vi "Example Graph.vi"() -> ()   [LabVIEW 2013]
uses:
  C:/tf/play/labview/Tinkerforge.dll
  Tinkerforge.dll
panel:
  in  "semsor identifier":u8=179
  in  "stop":bool
  out "graph":sgl[](graph)
  in  "uid":string="Fax"
  in  "port":i32=4223
  in  "host":string="localhost"
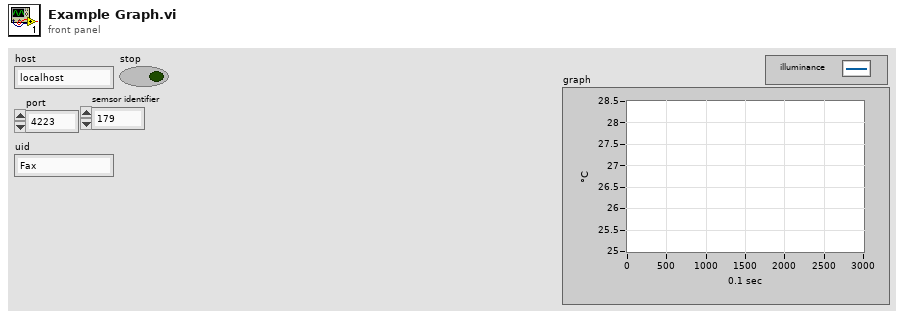
[diagram p1: front panel]
types:
  T1 = cluster{"humidity":u8, "identifier":u8, "temperature":i16}
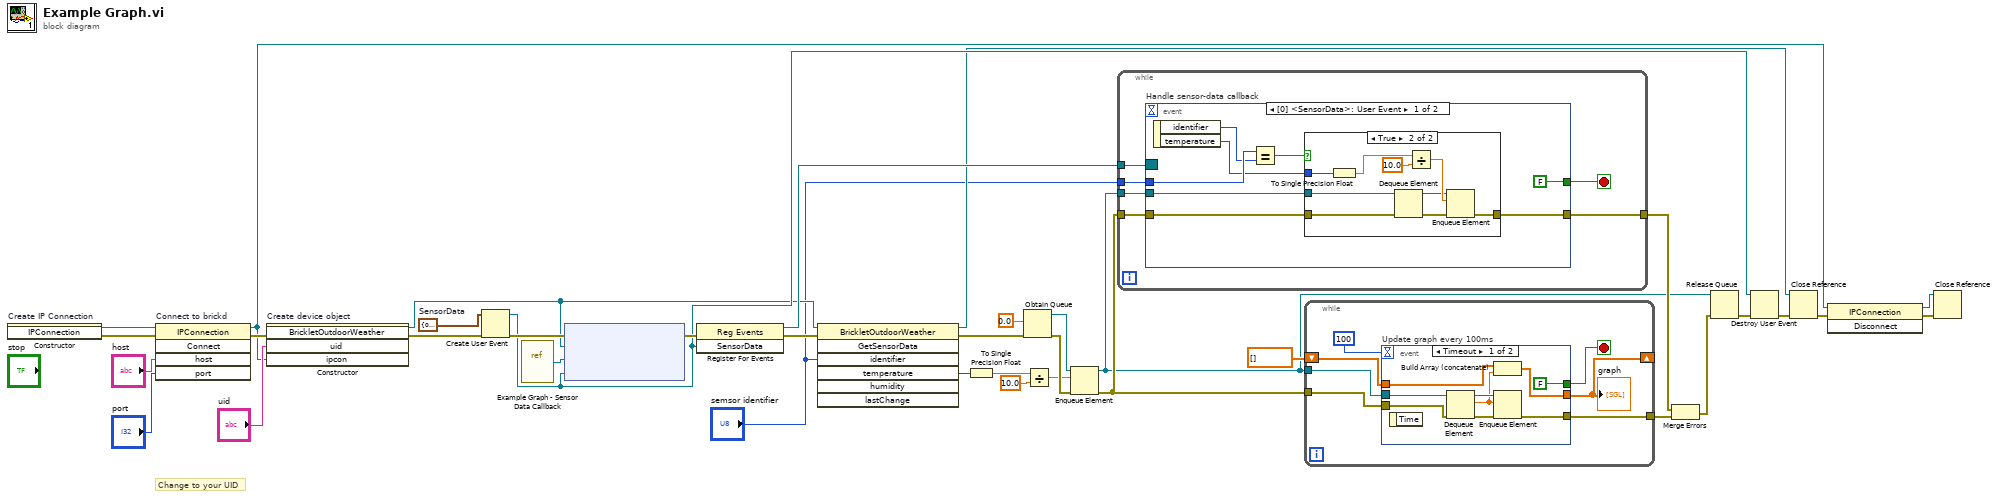
[diagram p0: block diagram]
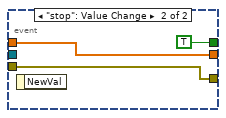
[diagram p2: hidden frame]
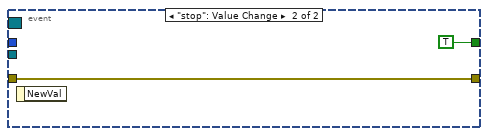
[diagram p4: hidden frame]
diagram:
  w23 = T1 {"humidity"=0, "identifier"=0, "temperature"=0}  # SensorData
  # "Change to your UID"
  n1 = constructor on="Create IP Connection" class="IPConnection"() -> (reference out=w37:refnum<k24>, error out=w12:errorcluster)  [unwired: 3 in, 1 out]
  n2 = invoke on="Connect to brickd" class="IPConnection" method="Connect"(reference=w37, error in=w12, "host"="host", "port"="port") -> (reference out=w30:refnum<k24>, error out=w33:errorcluster)  [unwired: 1 in, 3 out]
  n3 = constructor on="Create device object" class="BrickletOutdoorWeather"(error in=w33, "uid"="uid", "ipcon"=w30) -> (reference out=w6:refnum<k24>, error out=w5:errorcluster)  [unwired: 2 in, 3 out]
  n4 = Create User Event(user event datatype=w23, error in=w5) -> (user event=w25:refnum<user-event>, error out=w28:errorcluster)
  n5 = vi-ref "Example Graph - Sensor Data Callback.vi"() -> ("vi reference"=w4:refnum<vi>)
  n6 = node ("Register Event Callback")(w28, w6, w4, w25) -> (w27:errorcluster)  [unwired: 1 in, 1 out]
  n7 = register-events(error in=w27, w25) -> (reference out=w26:refnum<event-registration>, error out=w11:errorcluster)  [unwired: 1 in]
  n8 = invoke class="BrickletOutdoorWeather" method="GetSensorData"(reference=w6, error in=w11, "identifier"="semsor identifier") -> (reference out=w9:refnum<k24>, error out=w10:errorcluster, "temperature"=w2:i16)  [unwired: 4 in, 4 out]
  n9 = To Single Precision Float(number=w2) -> (single precision float=w1:sgl)
  n10 = Obtain Queue(element data type=sgl 0.0, error in (no error)=w10) -> (queue out=w16:refnum<queue>, error out=w18:errorcluster)  [unwired: 3 in, 1 out]
  n11 = Divide(x=w1, y=sgl 10.0) -> (x/y=w7:sgl)
  n12 = Enqueue Element(queue=w16, element=w7, error in (no error)=w18) -> (queue out=w13:refnum<queue>, error out=w17:errorcluster)  [unwired: 1 in, 1 out]
  n13 = while {
    tunnel: w26 -> [w43]
    tunnel: [w41] -> w21
    tunnel: w17 -> [w42]
    tunnel: w13 -> [w40]
    tunnel: "semsor identifier" -> [w38]
    stop <- w39 stop-if-true
    n14 = event "Handle sensor-data callback" shown="[0] <SensorData>: User Event" {
      selector: w43 -> [_ _]
      dyn-events: _ -> [_ _]
      timeout: _ -> [_ _]
      tunnel: w42 -> [w45 w62]
      tunnel: [w44 w62] -> w41
      tunnel: w40 -> [w46 _]
      tunnel: [FALSE TRUE] -> w39
      tunnel: w38 -> [w50 _]
      event User Event {
        n15 = event-data() -> ("identifier"=w49:u8, "temperature"=w47:i16)  [unwired: 1 in]
        n16 = Equal?(x=w50, y=w49) -> (x = y?=w48:bool)
        n17 = case shown="True" w48 {
          tunnel: w47 -> [_ w61]
          tunnel: w46 -> [_ w55]
          tunnel: w45 -> [w52 w54]
          tunnel: [w52 w53] -> w44
          frame False {
          }
          frame True {
            n18 = To Single Precision Float(number=w61) -> (single precision float=w56:sgl)
            n19 = Dequeue Element(queue=w55, error in (no error)=w54) -> (queue out=w59:refnum<queue>, error out=w58:errorcluster)  [unwired: 1 in, 2 out]
            n20 = Divide(x=w56, y=sgl 10.0) -> (x/y=w60:sgl)
            n21 = Enqueue Element(queue=w59, element=w60, error in (no error)=w58) -> (error out=w53:errorcluster)  [unwired: 1 in, 2 out]
          }
        }
      }
      event "stop": Value Change {
        n22 = event-data() -> ()  [unwired: 1 in, 1 out]
      }
    }
  }
  n23 = while {
    tunnel: [w66] -> w22
    tunnel: w17 -> [w67]
    shift-right: [w68] -> _
    shift-left: sgl[] [] -> [w69]
    tunnel: w13 -> [w65]
    stop <- w64 stop-if-true
    n24 = event "Update graph every 100ms" shown="[0] Timeout" {
      selector: _ -> [_ _]
      dyn-events: _ -> [_ _]
      timeout: 100 -> [_ _]
      tunnel: [w79 w81] -> w68
      tunnel: w69 -> [w72 w81]
      tunnel: w67 -> [w78 w80]
      tunnel: [w75 w80] -> w66
      tunnel: w65 -> [w77 _]
      tunnel: [FALSE TRUE] -> w64
      event Timeout {
        n25 = event-data() -> ()  [unwired: 1 in, 1 out]
        n26 = Dequeue Element(queue=w77, error in (no error)=w78) -> (queue out=w74:refnum<queue>, element=w73:sgl, error out=w76:errorcluster)  [unwired: 1 in, 1 out]
        n27 = Build Array (concatenate)(w72, w73) -> (w79:sgl[])
        n28 = Enqueue Element(queue=w74, element=w73, error in (no error)=w76) -> (error out=w75:errorcluster)  [unwired: 1 in, 2 out]
      }
      event "stop": Value Change {
        n29 = event-data() -> ()  [unwired: 1 in, 1 out]
      }
    }
    "graph" <- w68
  }
  n30 = Merge Errors(w21, w22) -> (w15:errorcluster)
  n31 = Release Queue(queue=w13, error in (no error)=w15) -> (error out=w14:errorcluster)  [unwired: 1 in, 2 out]
  n32 = Destroy User Event(user event=w25, error in=w14) -> (error out=w24:errorcluster)
  n33 = Close Reference(reference=w9, error in (no error)=w24) -> (error out=w32:errorcluster)
  n34 = invoke class="IPConnection" method="Disconnect"(reference=w30, error in=w32) -> (reference out=w29:refnum<k24>, error out=w31:errorcluster)  [unwired: 1 in, 1 out]
  n35 = Close Reference(reference=w29, error in (no error)=w31) -> ()  [unwired: 1 out]
